vi "ALTS-2015 Enqueue Unload Task State.vi"(8 "error in (no error)":errorcluster, 11 "Unload Tasks In":T1[](array[typedef])) -> (0 "error out":errorcluster, 3 "Unload Tasks Out":T1[](array[typedef]))   [LabVIEW 2013]
uses:
  Controls/ALTS-2015 Unload Task Data.ctl
  Controls/ALTS-2015 Station Cluster.ctl
  Controls/ALTS-2015 LV2GBL Station Info Options.ctl
  Controls/ALTS-2015 Ring Indicator Enum.ctl
  Controls/ALTS-2015 Status Ring Indicator.ctl
  Controls/ALTS-2015 Station Details.ctl
  Controls/ALTS-2015 Robot Actions.ctl
  Controls/ALTS-2015 Robot Tasks.ctl
  Controls/ALTS-2015 Robot FIFO Queue Options.ctl
  Controls/ALTS-2015 Serial Details.ctl
  Controls/ALTS-2015 Serial DB Details.ctl
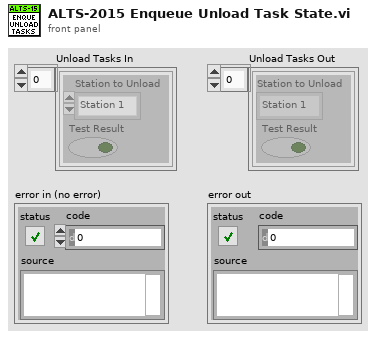
[diagram p1: front panel]
types:
  T1 = typedef "ALTS-2015 Unload Task Data.ctl" = cluster{"Station to Unload":T2, "Test Result":bool}
  T2 = typedef "ALTS-2015 Station Cluster.ctl" = enum16{"Station 1", "Station 2", "Station 3", "Station 4"}
  T3 = typedef "ALTS-2015 Status Ring Indicator.ctl" = u16
  T4 = typedef "ALTS-2015 Ring Indicator Enum.ctl" = enum16{"Idle", "Test Running", "Unit Clamped", "Unit not Clamped", "Pass", "Fail"}
  T5 = typedef "ALTS-2015 LV2GBL Station Info Options.ctl" = enum16{"Init", "Read", "Read All", "Write Sensor ID", "Write  Work Order", "Write Serial Number", "Write Test Data", "Write Station Status", "Write Station Occupancy", "Write Station Test Type", "Write Rerun", "Write Load Decision", "Write Robot Action", "Clear All", "Clear Test Result"}
  T6 = typedef "ALTS-2015 Robot FIFO Queue Options.ctl" = enum16{"Init", "Enqueue", "Dequeue", "Get Queue Elements", "Flush", "Destroy"}
  T7 = typedef "ALTS-2015 Robot Tasks.ctl" = enum16{"Load", "Unload", "Rerun", "Invalid Serial"}
  T8 = typedef "ALTS-2015 Station Details.ctl" = cluster{"Station Number":string, "Work Order Number":string, "Sensor Name":string, "Pressure (PSI)":string, "Flow (SCCM)":string, "Test Time ":string, "Test Result":string, "Serial Number":string, "Station Status":T3, "SW assigned UUT":bool, "Rerun Count":i32, "Test Type":i32, "Load Decision":i32, "Robot Action":T9}
  T9 = typedef "ALTS-2015 Robot Actions.ctl" = enum16{"Loading...", "Unloading...", "Reruning...", "No Action"}
  T10 = typedef "ALTS-2015 Serial Details.ctl" = cluster{"Robot Task":T7, "Serial No":string, "New Serial?":bool, "Station # Unload":T2, "Last Test Result":bool, "Rerun?":bool, "Station # Rerun":T2, "Invalid Serial?":bool, "Serial Details":T11}
  T11 = typedef "ALTS-2015 Serial DB Details.ctl" = cluster{"Adapter Plate Size":i32, "Air Leak Test Type ":i32, "Displacement Size":i32, "Flange Size":i32, "Height":i32, "Load Decision":i32, "Cart Insert":i32}
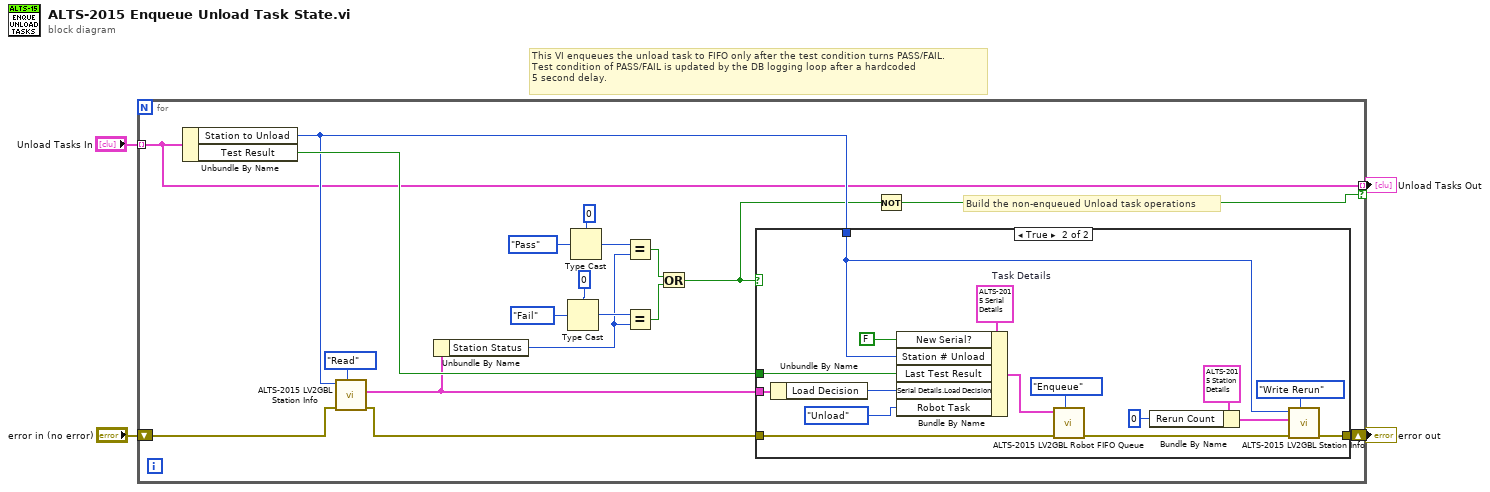
[diagram p0: block diagram]
diagram:
  # "This VI enqueues the unload task to FIFO only after the test condition turns PASS/FAIL.\nTest condition of PASS/FAIL is updated by the DB logging loop after a hardcoded\n5 second delay."
  n1 = for {
    tunnel: "Unload Tasks In" -> [w17] mode=indexing
    shift-right: [w23] -> w2
    shift-left: "error in (no error)" -> [w20]
    tunnel: [w17] -> w4 mode=indexing if=w10
    # "Build the non-enqueued Unload task operations"
    n2 = Unbundle By Name(w17) -> ("Station to Unload"=w18:T2, "Test Result"=w22:bool)
    n3 = call "ALTS-2015 LV2GBL Station Info.vi"("Options"=ALTS-2015_LV2GBL_Station_Info_Options."Read", "error in"=w20, "Station Cluster"=w18) -> ("error out"=w19:errorcluster, "Station Details"=w9:T8)  [unwired: 6 in, 1 out]
    n4 = Unbundle By Name(w9) -> ("Station Status"=w8:T3)
    n5 = Type Cast(type=T3 0 ("Station Status"), x=ALTS-2015_Ring_Indicator_Enum."Fail" ("Ring Indicator Options")) -> (*(type *) &x=w13:T3)
    n6 = Type Cast(type=T3 0 ("Station Status"), x=ALTS-2015_Ring_Indicator_Enum."Pass" ("Ring Indicator Options")) -> (*(type *) &x=w14:T3)
    n7 = Equal?(x=w14, y=w8) -> (x = y?=w12:bool)
    n8 = Equal?(x=w13, y=w8) -> (x = y?=w11:bool)
    n9 = Or(x=w12, y=w11) -> (x .or. y?=w5:bool)
    n10 = case shown="True" w5 {
      tunnel: [w24 w40] -> w23
      tunnel: w22 -> [_ w39]
      tunnel: w19 -> [w24 w38]
      tunnel: w18 -> [_ w37]
      tunnel: w9 -> [_ w31]
      frame False {
      }
      frame True {
        w27 = T10 {"Robot Task"=enum."Load", "Serial No"="", "New Serial?"=FALSE, "Station # Unload"=enum."Station 1", "Last Test Result"=FALSE, "Rerun?"=FALSE, "Station # Rerun"=enum."Station 1", "Invalid Serial?"=FALSE, "Serial Details"={"Adapter Plate Size"=0, "Air Leak Test Type "=0, "Displacement Size"=0, "Flange Size"=0, "Height"=0, "Load Decision"=0, "Cart Insert"=0}}  # Task Details
        n11 = Unbundle By Name(w31) -> ("Load Decision"=w29:i32)
        n12 = Bundle By Name(cluster=w27, "New Serial?"=FALSE ("New Part?"), "Station # Unload"=w37, "Last Test Result"=w39, "Serial Details.Load Decision"=w29, "Robot Task"=ALTS-2015_Robot_Tasks."Unload") -> (w25:T10)
        n13 = call "ALTS-2015 LV2GBL Robot FIFO Queue.vi"("Options"=ALTS-2015_Robot_FIFO_Queue_Options."Enqueue" ("Enum"), "error in (no error)"=w38, "Task Details In"=w25) -> ("error out"=w32:errorcluster)  [unwired: 4 in, 4 out]
        n14 = Bundle By Name(cluster=T8 {"Station Number"="", "Work Order Number"="", "Sensor Name"="", "Pressure (PSI)"="", "Flow (SCCM)"="", "Test Time "="", "Test Result"="", "Serial Number"="", "Station Status"=0, "SW assigned UUT"=FALSE, "Rerun Count"=0, "Test Type"=0, "Load Decision"=0, "Robot Action"=enum."Loading..."} ("Station"), "Rerun Count"=0) -> (w35:T8)
        n15 = call "ALTS-2015 LV2GBL Station Info.vi"("Options"=ALTS-2015_LV2GBL_Station_Info_Options."Write Rerun", "error in"=w32, "Station"=w35, "Station Cluster"=w37) -> ("error out"=w40:errorcluster)  [unwired: 5 in, 2 out]
      }
    }
    n16 = Not(x=w5) -> (.not. x?=w10:bool)
  }
  "Unload Tasks Out" <- w4
  "error out" <- w2
